vi "Controller Acquisition and Actuation Loop.vi"(4 "Iteration duration":u64, 5 "Missed iteration count":u32, 6 "Timestamp":u64, 7 "Sync Objects":T3, 8 "error in (no error)":errorcluster, 9 "PS Variables":T1, 10 "BPM Variables":T2, 11 "FOFB Configuration":T6={"FOFB Parameters"={"Network"={"FOFB Controller IP"="", "LNLS Control Network IP"="", "LNLS Control Network Power Supplies TCP Port"=0, "LNLS Control Network FOFB Configuration TCP Port"=0, "LNLS Control Network BPMs TCP Port"=0, "Data Server TCP Port"=0, "Monitoring Data TCP Port"=0, "Configuration GUI TCP Port"=0, "Storage Data TCP Port"=0, "Fast Command TCP Port"=0, "TCP Listening Timeout"=0, "Request Setpoints Rate"=0}, "Fast Acquisition"={"Acquisition Period"=0, "Data Buffer Size"=0, "Monitoring Period"=0}, "Response Matrix Measurement"={"Step Amplitude"=0.0, "Time Between Steps"=0, "Step Duration"=0, "Number of Averages"=0}, "Correction Algorithm"={"Correction Period"=0, "Reference Orbit Path"=path "", "Response Matrix Path"=path "", "Correction Matrix Path"=path "", "PID Horizontal Gain"=0.0, "PID Vertical Gain"=0.0, "PID Horizontal Integral Time"=0.0, "PID Vertical Integral Time"=0.0, "PID Horizontal Derivative Time"=0.0, "PID Vertical Derivative Time"=0.0, "Beam Current FOFB Threshold"=0.0, "Decouple H-V"=FALSE, "Use Additional BPM LPF"=FALSE, "BPM LPF Cutoff"=0.0}, "Acquisition Network"=[], "Actuation Network"=[]}, "Number of Acquisition Chassis"=0, "Number of Actuation Chassis"=0, "Number of BPM Readings"=0, "BPM Reading Names"=[], "Selected BPM Readings"=[0, 1, 2, 3, 4, 5, 6, 7, 8, 9, 10, 11, 12, 13, 14, 15, 16, 17, 18, 19, 20, 21, 22, 23, 24, 25, 26, 27, 28, 29, 30, 31, 32, 33, 34, 35, 36, 37, 38, 39, 40, 41, 42, 43, 44, 45, 46, 47, 48, 49], "Number of Correctors"=0, "Corrector Names"=[], "Selected Correctors"=[0, 1, 2, 3, 4, 5, 6, 7, 8, 9, 10, 11, 12, 13, 14, 15, 16, 17, 18, 19, 20, 21, 22, 23, 24, 25, 26, 27, 28, 29, 30, 31, 32, 33, 34, 35, 36, 37, 38, 39, 40, 41, 42, 43, 44, 45, 46, 47, 48, 49], "Reference Orbit"=[], "Response Matrix"=[], "Correction Matrix"=[], "Acquisition Chassis Names"=[], "Actuation Chassis Names"=[], "Acquisition Variables"=[], "Actuation Variables"=[], "PS Matrix Mapping"=[], "Inverse PS Matrix Mapping"=[], "BPM Matrix Mapping"=[], "Inverse BPM Matrix Mapping"=[], "Response Matrix Beam Energy (MeV)"=0.0, "PID Parameters"=[], "BPM Planes"=[], "Corrector Planes"=[], "RMM Step Factor"=[]}) -> (0 "error out":errorcluster)   [LabVIEW 2011, in "Controller VIs.lvlib"]
doc: "Continuously performs acquisition of all input variables (BPM readings, Power Supply readings, etc.) and forwards data to the <b>Decimated Acquisition Loop</b>. Depending on the <b>Actuation State</b> (global variable), performs actuations coming from one of the following sources (global variables):\n\n<b>Actuation State</b> = Only Reading\n (no actuation)\n\n<b>Actuation State</b> = Manual\n PS_Manual_Setpoints\n\n<b>Actuation State</b> = FOFB, Initializing FOFB, Stopping FOFB\n PS_FOFB_Setpoints\n\n<b>Actuation State</b> = Response Matrix Measurement\n PS_RMM_Setpoints"
uses:
  Controller VIs.lvlib
  Types Definitions/Type FOFB Configuration.ctl
  Types Definitions/Type FOFB Parameters.ctl
  Types Definitions/Type Network Configuration.ctl
  Types Definitions/Type FA Configuration.ctl
  Types Definitions/Type Response Matrix Measurement Configuration.ctl
  Types Definitions/Type Correction Algorithm Configuration.ctl
  Types Definitions/Type Acquisition Network Configuration.ctl
  Types Definitions/Type Actuation Network Configuration.ctl
  Types Definitions/Type PID Parameters.ctl
  Types Definitions/Type Synchronization Objects.ctl
  Types Definitions/Type Blocking Synchronization Objects.ctl
  Types Definitions/Type Monitoring Data.ctl
  Types Definitions/Type Operation Mode State.ctl
  Types Definitions/Type Diagnostics Data.ctl
  Types Definitions/Type CPU Loads Array.ctl
  Types Definitions/Type CPU Loads.ctl
  Types Definitions/Type Non-blocking Synchronization Objects.ctl
  Types Definitions/Type FOFB Variables.ctl
  Types Definitions/Type Actuation State.ctl
  Types Definitions/Type BPM Variables.ctl
  Types Definitions/Type PS Variables.ctl
  Controller Write FXP20.5.vi
  Controller Global Variables/Controller Actuation State.vi
  Type Definitions.lvlib
  Controller Global Variables.lvlib
panel:
  in  "Numeric":i32=3125
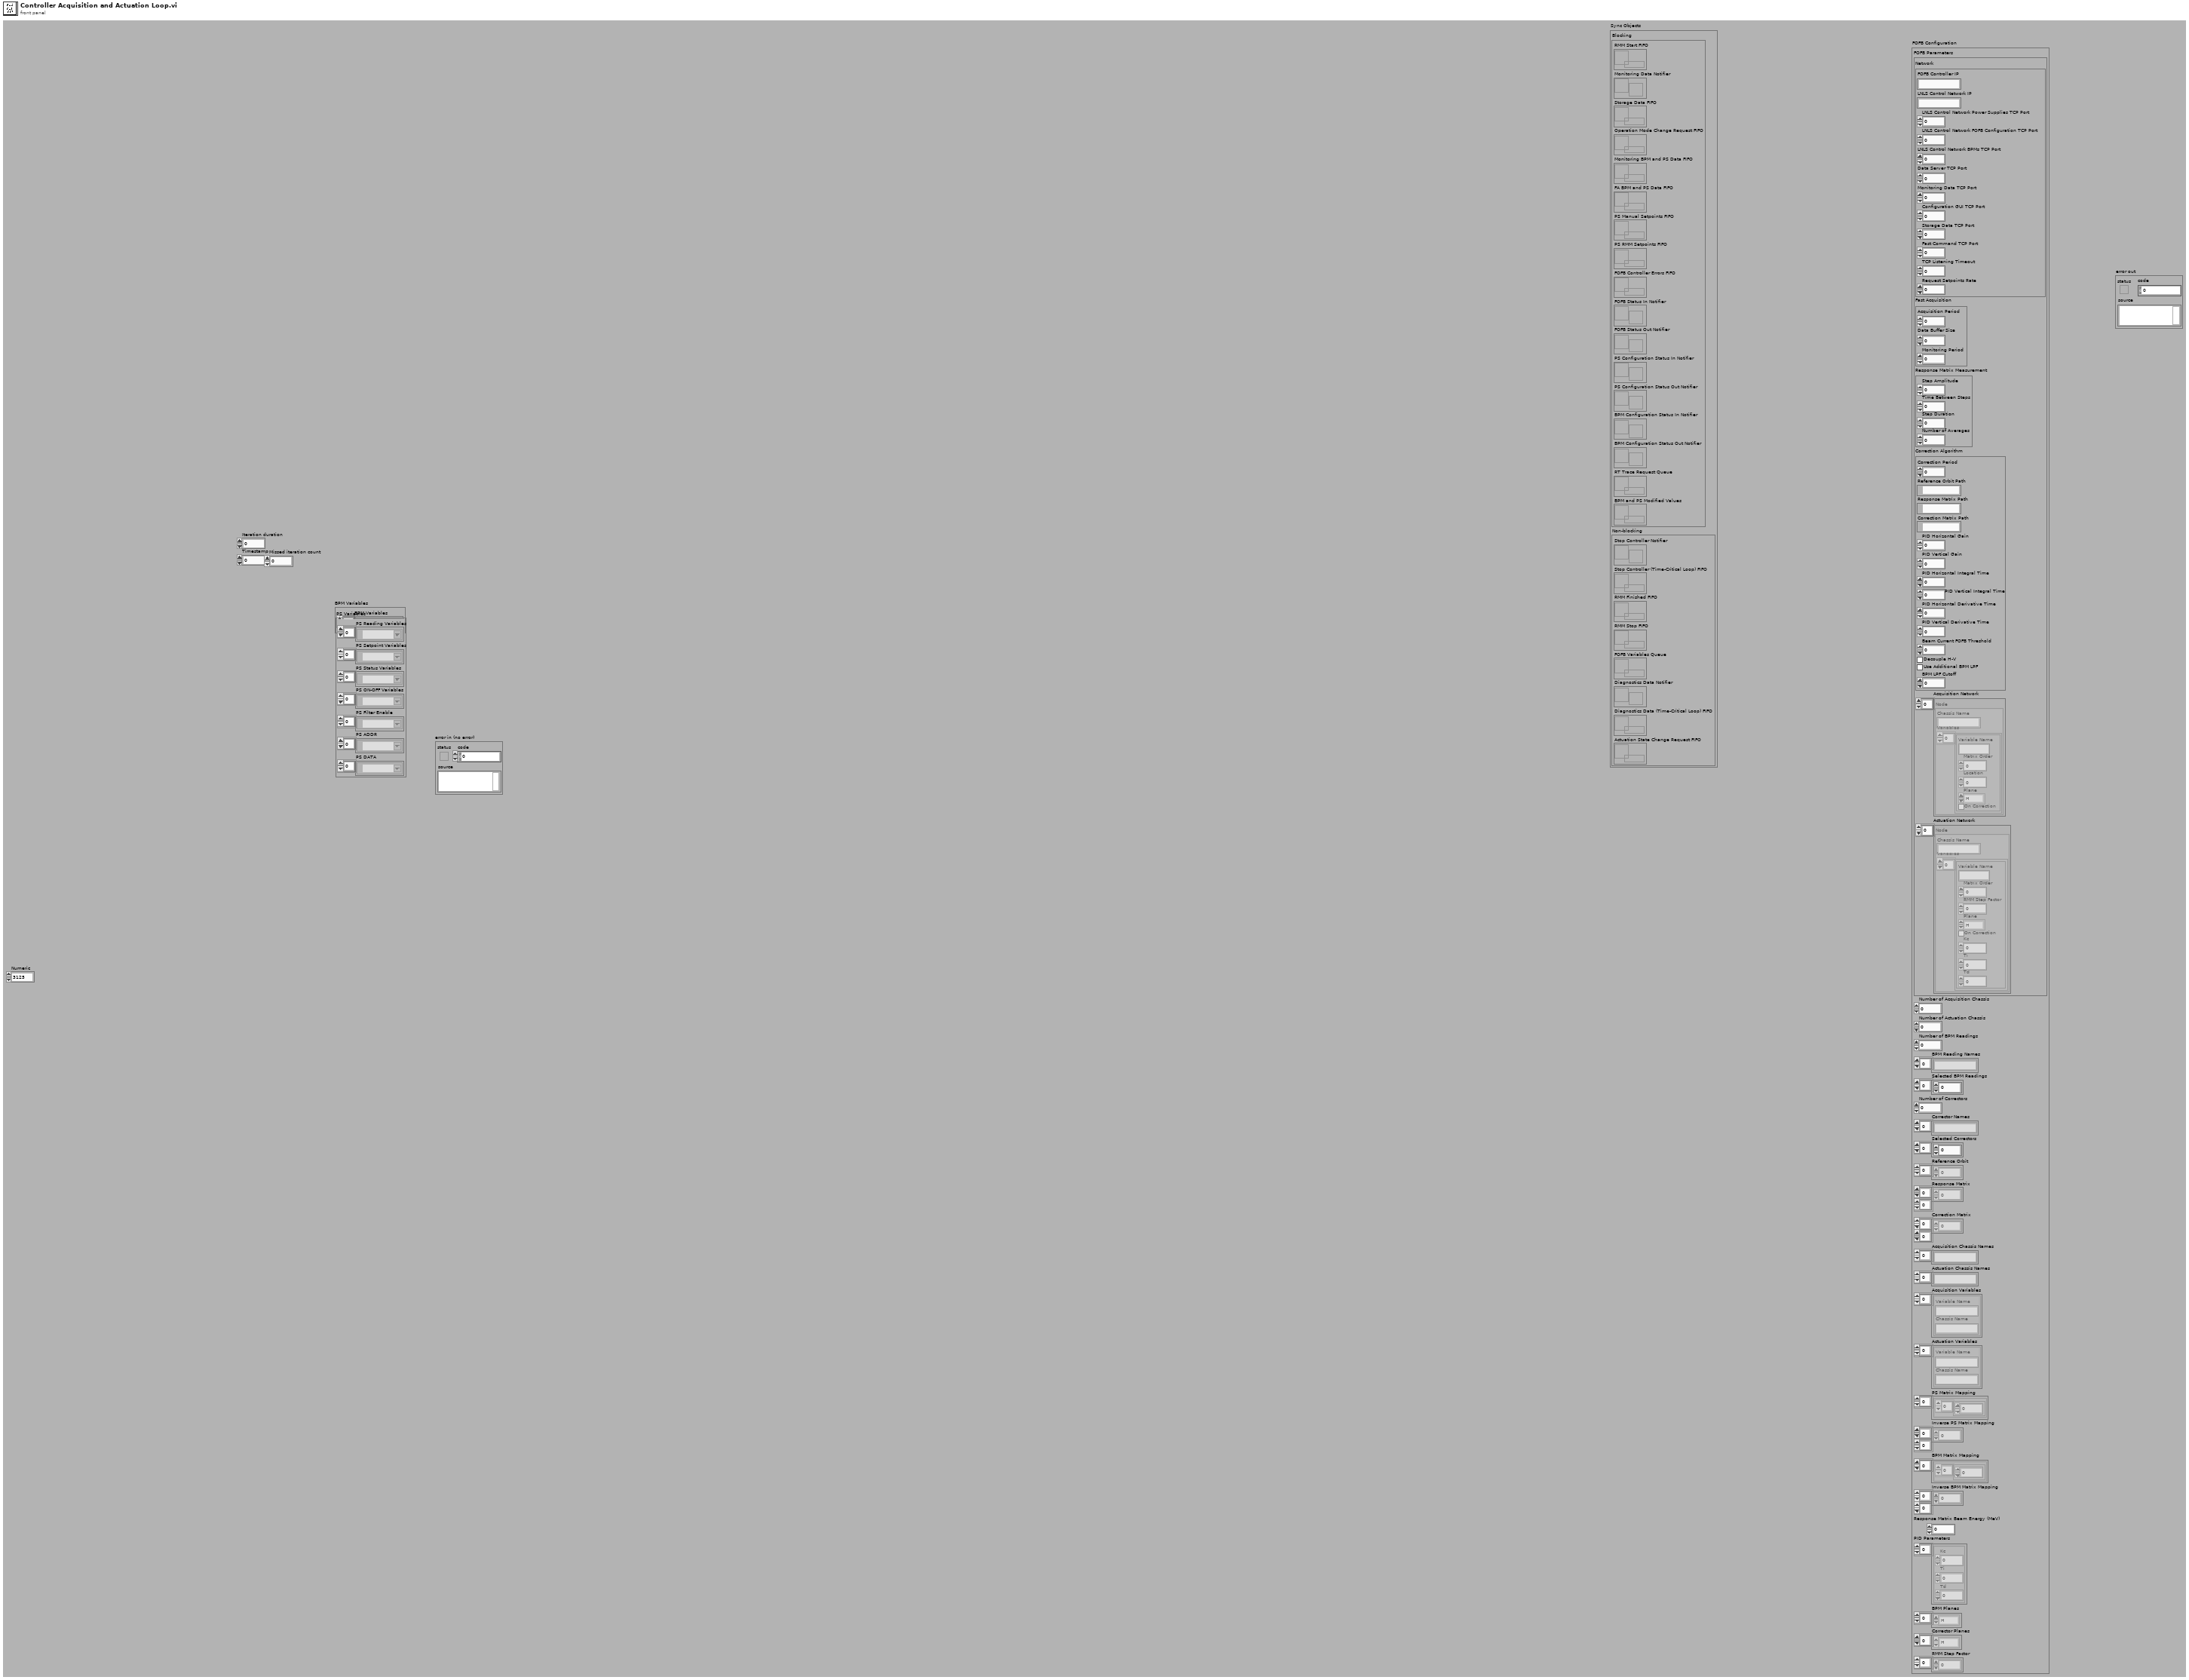
[diagram p1: front panel]
types:
  T1 = typedef "Type Definitions.lvlib/Type PS Variables.ctl" = cluster{"PS Reading Variables":refnum<k21>[], "PS Setpoint Variables":refnum<k21>[], "PS Status Variables":refnum<k21>[], "PS ON-OFF Variables":refnum<k21>[], "PS Filter Enable":refnum<k21>[], "PS ADDR":refnum<k21>[], "PS DATA":refnum<k21>[]}
  T2 = typedef "Type Definitions.lvlib/Type BPM Variables.ctl" = cluster{"BPM Variables":refnum<k21>[]}
  T3 = typedef "Type Definitions.lvlib/Type Synchronization Objects.ctl" = cluster{"Blocking":T4, "Non-blocking":T5}
  T4 = typedef "Type Definitions.lvlib/Type Blocking Synchronization Objects.ctl" = cluster{"RMM Start FIFO":refnum<k33>, "Monitoring Data Notifier":refnum<notifier>, "Storage Data FIFO":refnum<queue>, "Operation Mode Change Request FIFO":refnum<k33>, "Monitoring BPM and PS Data FIFO":refnum<k33>, "FA BPM and PS Data FIFO":refnum<k33>, "PS Manual Setpoints FIFO":refnum<k33>, "PS RMM Setpoints FIFO":refnum<k33>, "FOFB Controller Errors FIFO ":refnum<k33>, "FOFB Status In Notifier":refnum<notifier>, "FOFB Status Out Notifier":refnum<notifier>, "PS Configuration Status In Notifier":refnum<notifier>, "PS Configuration Status Out Notifier":refnum<notifier>, "BPM Configuration Status In Notifier":refnum<notifier>, "BPM Configuration Status Out Notifier":refnum<notifier>, "RT Trace Request Queue":refnum<queue>, "BPM and PS Modified Values":refnum<k33>}
  T5 = typedef "Type Definitions.lvlib/Type Non-blocking Synchronization Objects.ctl" = cluster{"Stop Controller Notifier":refnum<notifier>, "Stop Controller (Time-Critical Loop) FIFO":refnum<k33>, "RMM Finished FIFO":refnum<k33>, "RMM Stop FIFO":refnum<k33>, "FOFB Variables Queue":refnum<queue>, "Diagnostics Data Notifier":refnum<notifier>, "Diagnostics Data (Time-Critical Loop) FIFO":refnum<k33>, "Actuation State Change Request FIFO":refnum<k33>}
  T6 = typedef "Type Definitions.lvlib/Type FOFB Configuration.ctl" = cluster{"FOFB Parameters":T7, "Number of Acquisition Chassis":i32, "Number of Actuation Chassis":i32, "Number of BPM Readings":i32, "BPM Reading Names":string[], "Selected BPM Readings":u32[], "Number of Correctors":i32, "Corrector Names":string[], "Selected Correctors":u32[], "Reference Orbit":dbl[], "Response Matrix":dbl[][], "Correction Matrix":dbl[][], "Acquisition Chassis Names":string[], "Actuation Chassis Names":string[], "Acquisition Variables":cluster{"Variable Name":string, "Chassis Name":string}[], "Actuation Variables":cluster{"Variable Name":string, "Chassis Name":string}[], "PS Matrix Mapping":cluster{u32[]}[], "Inverse PS Matrix Mapping":u32[][], "BPM Matrix Mapping":cluster{u32[]}[], "Inverse BPM Matrix Mapping":u32[][], "Response Matrix Beam Energy (MeV)":dbl, "PID Parameters":T14[], "BPM Planes":enum8{"H", "V"}[], "Corrector Planes":enum8{"H", "V"}[], "RMM Step Factor":dbl[]}
  T7 = typedef "Type Definitions.lvlib/Type FOFB Parameters.ctl" = cluster{"Network":T8, "Fast Acquisition":T9, "Response Matrix Measurement":T10, "Correction Algorithm":T11, "Acquisition Network":T12, "Actuation Network":T13}
  T8 = typedef "Type Definitions.lvlib/Type Network Configuration.ctl" = cluster{"FOFB Controller IP":string, "LNLS Control Network IP":string, "LNLS Control Network Power Supplies TCP Port":u16, "LNLS Control Network FOFB Configuration TCP Port":u16, "LNLS Control Network BPMs TCP Port":u16, "Data Server TCP Port":u16, "Monitoring Data TCP Port":u16, "Configuration GUI TCP Port":u16, "Storage Data TCP Port":u16, "Fast Command TCP Port":u16, "TCP Listening Timeout":i32, "Request Setpoints Rate":u16}
  T9 = typedef "Type Definitions.lvlib/Type FA Configuration.ctl" = cluster{"Acquisition Period":u32, "Data Buffer Size":u32, "Monitoring Period":u32}
  T10 = typedef "Type Definitions.lvlib/Type Response Matrix Measurement Configuration.ctl" = cluster{"Step Amplitude":dbl, "Time Between Steps":u32, "Step Duration":u32, "Number of Averages":u32}
  T11 = typedef "Type Definitions.lvlib/Type Correction Algorithm Configuration.ctl" = cluster{"Correction Period":u32, "Reference Orbit Path":path, "Response Matrix Path":path, "Correction Matrix Path":path, "PID Horizontal Gain":dbl, "PID Vertical Gain":dbl, "PID Horizontal Integral Time":dbl, "PID Vertical Integral Time":dbl, "PID Horizontal Derivative Time":dbl, "PID Vertical Derivative Time":dbl, "Beam Current FOFB Threshold":dbl, "Decouple H-V":bool, "Use Additional BPM LPF":bool, "BPM LPF Cutoff":dbl}
  T12 = typedef "Type Definitions.lvlib/Type Acquisition Network Configuration.ctl" = cluster{"Chassis Name":string, "Variables":cluster{"Variable Name":string, "Matrix Order":u32, "Location":dbl, "Plane":enum8{"H", "V"}, "On Correction":bool}[]}[]
  T13 = typedef "Type Definitions.lvlib/Type Actuation Network Configuration.ctl" = cluster{"Chassis Name":string, "Variables":cluster{"Variable Name":string, "Matrix Order":u32, "RMM Step Factor":dbl, "Plane":enum8{"H", "V"}, "On Correction":bool, "Kc":dbl, "Ti":dbl, "Td":dbl}[]}[]
  T14 = typedef "Type Definitions.lvlib/Type PID Parameters.ctl" = cluster{"Kc":fxp<+/-,16,8>, "Ti":fxp<+/-,16,8>, "Td":fxp<+/-,16,8>}
  T15 = typedef "Type Definitions.lvlib/Type Actuation State.ctl" = enum8{"Only reading", "Manual", "FOFB Initialization", "FOFB", "FOFB Stopping", "RMM Initialization", "RMM", "RMM Stopping"}
  T16 = typedef "Type Definitions.lvlib/Type FOFB Variables.ctl" = cluster{"Correction Period":u32, "Reference Orbit":dbl[], "Response Matrix":dbl[][], "Correction Matrix":dbl[][], "Decouple H-V":bool, "PID Horizontal Gain":dbl, "PID Vertical Gain":dbl, "PID Horizontal Integral Time":dbl, "PID Vertical Integral Time":dbl, "PID Horizontal Derivative Time":dbl, "PID Vertical Derivative Time":dbl, "Selected BPM Readings":u32[], "Selected Correctors":u32[], "BPM Planes":enum8{"H", "V"}[], "Corrector Planes":enum8{"H", "V"}[], "Beam Current FOFB Threshold":dbl, "Response Matrix Beam Energy (MeV)":dbl, "Fast Command Enabled":bool}
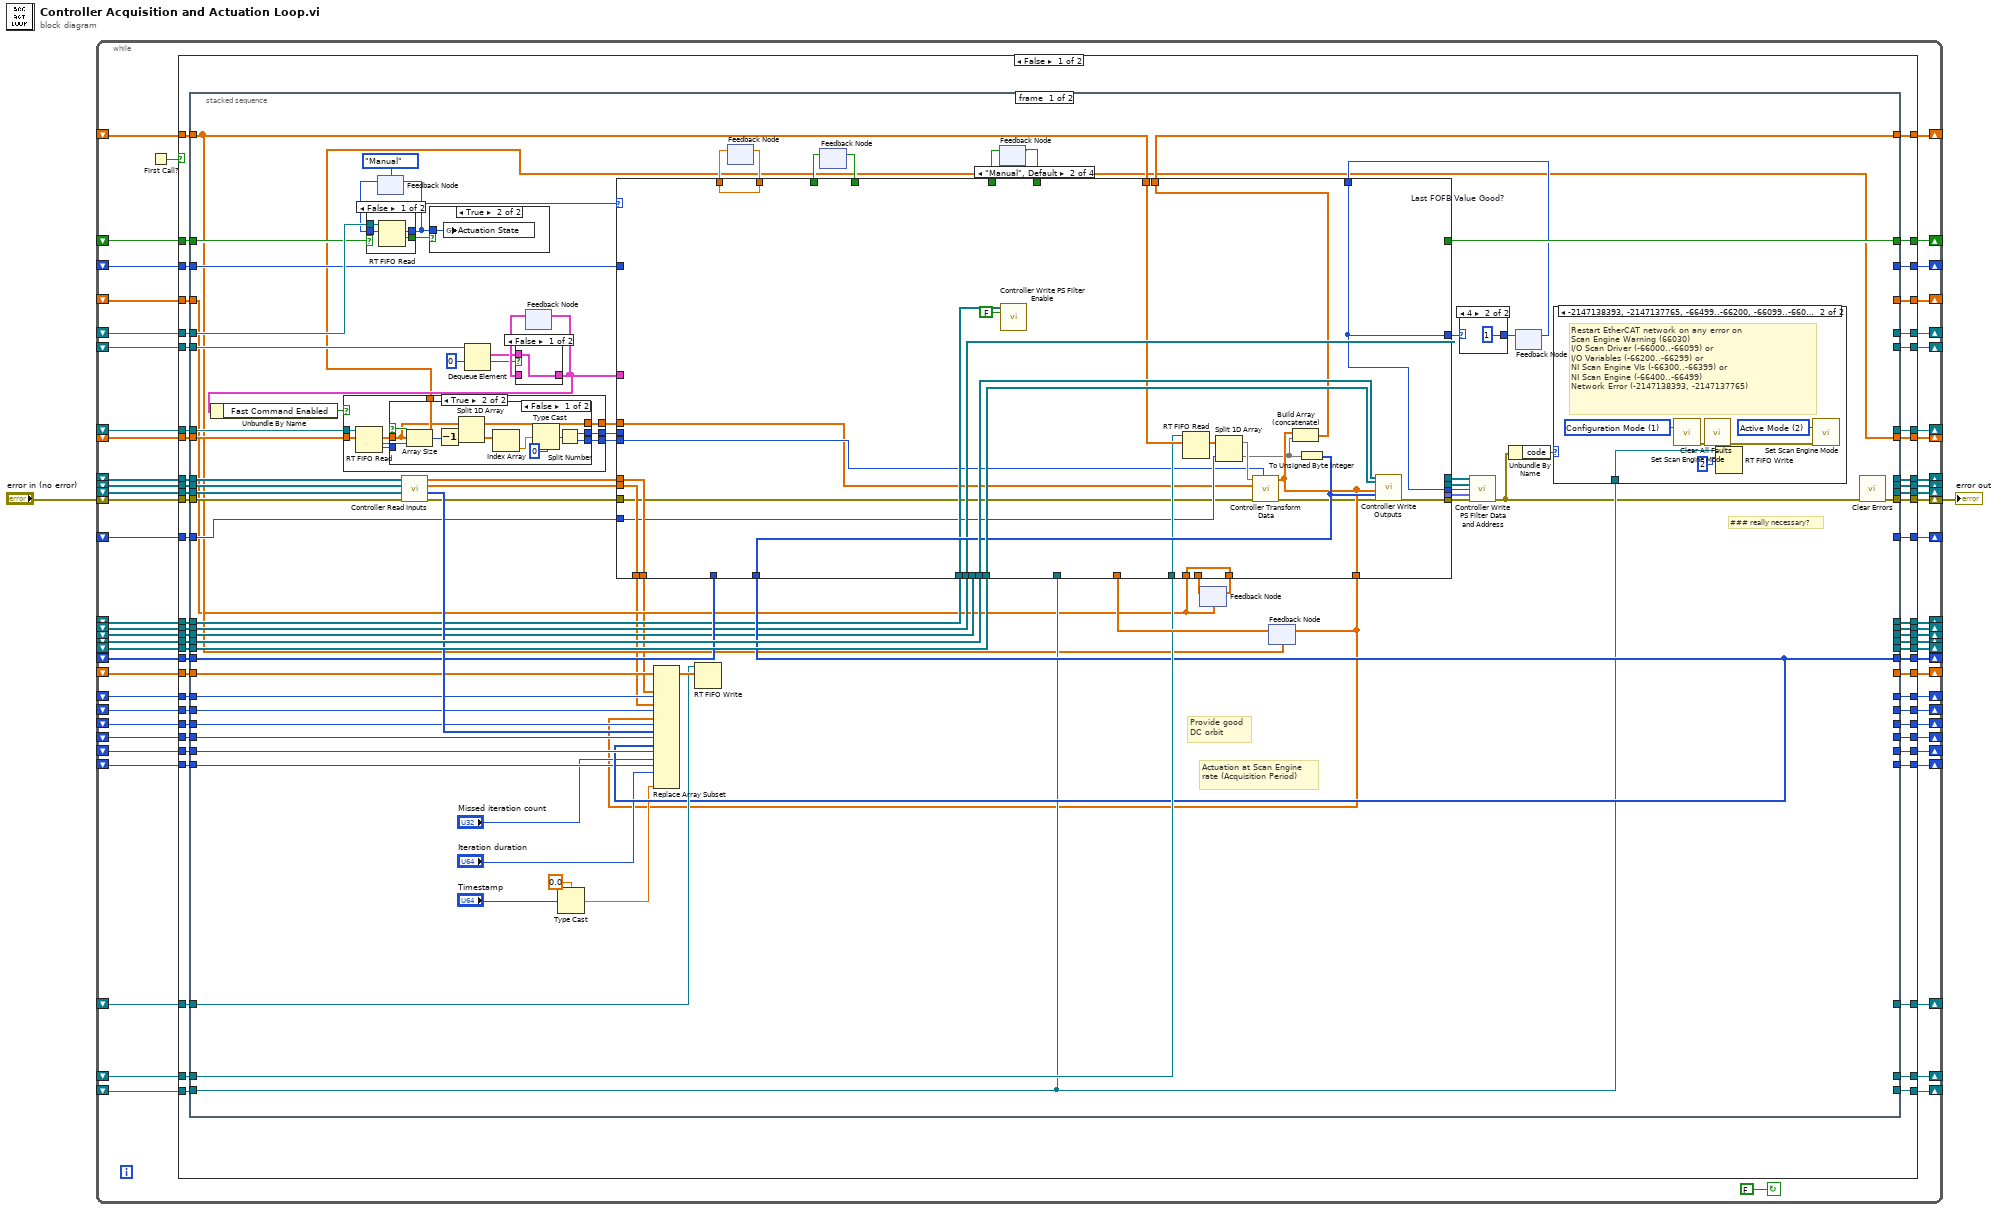
[diagram p0: block diagram]
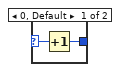
[diagram p3: hidden frame]
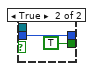
[diagram p4: hidden frame]
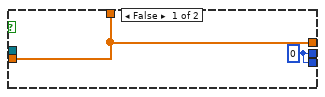
[diagram p5: hidden frame]
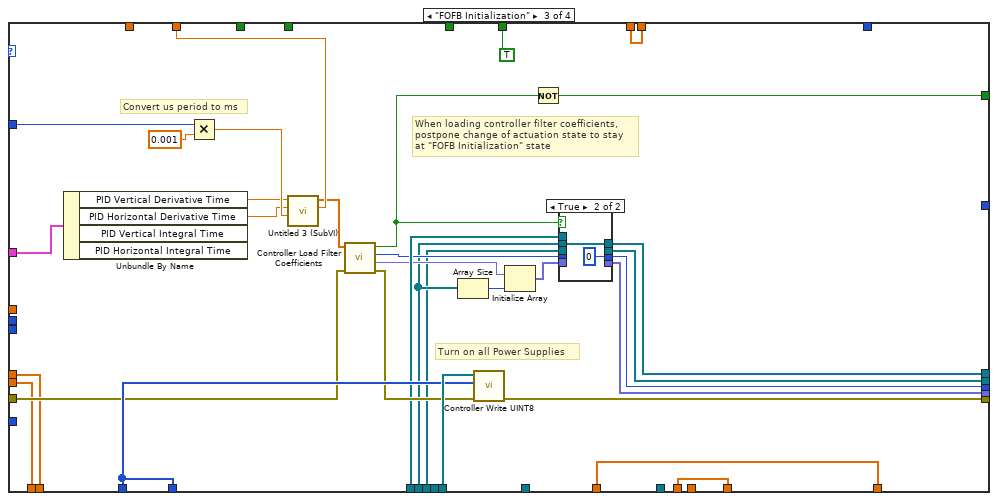
[diagram p10: hidden frame]
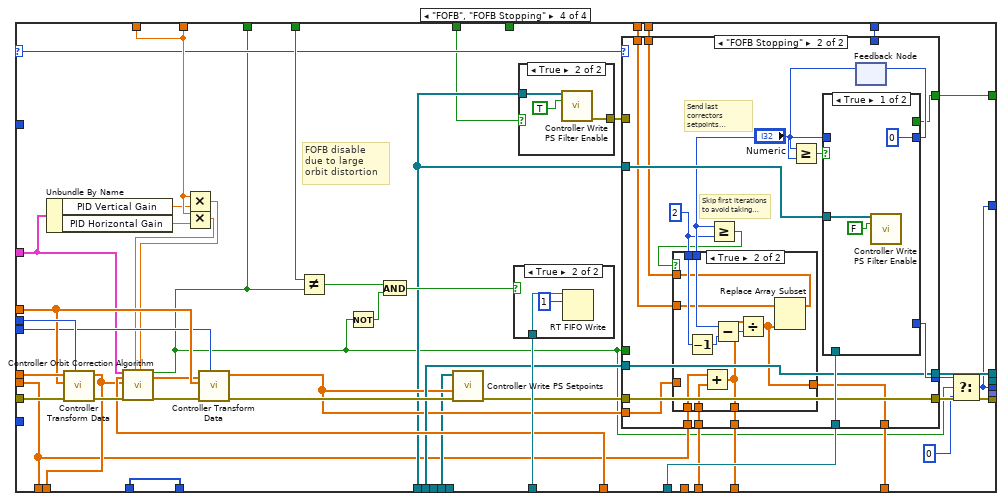
[diagram p12: hidden frame]
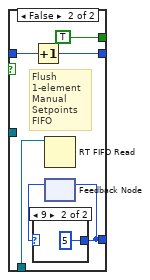
[diagram p15: hidden frame]
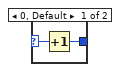
[diagram p16: hidden frame]
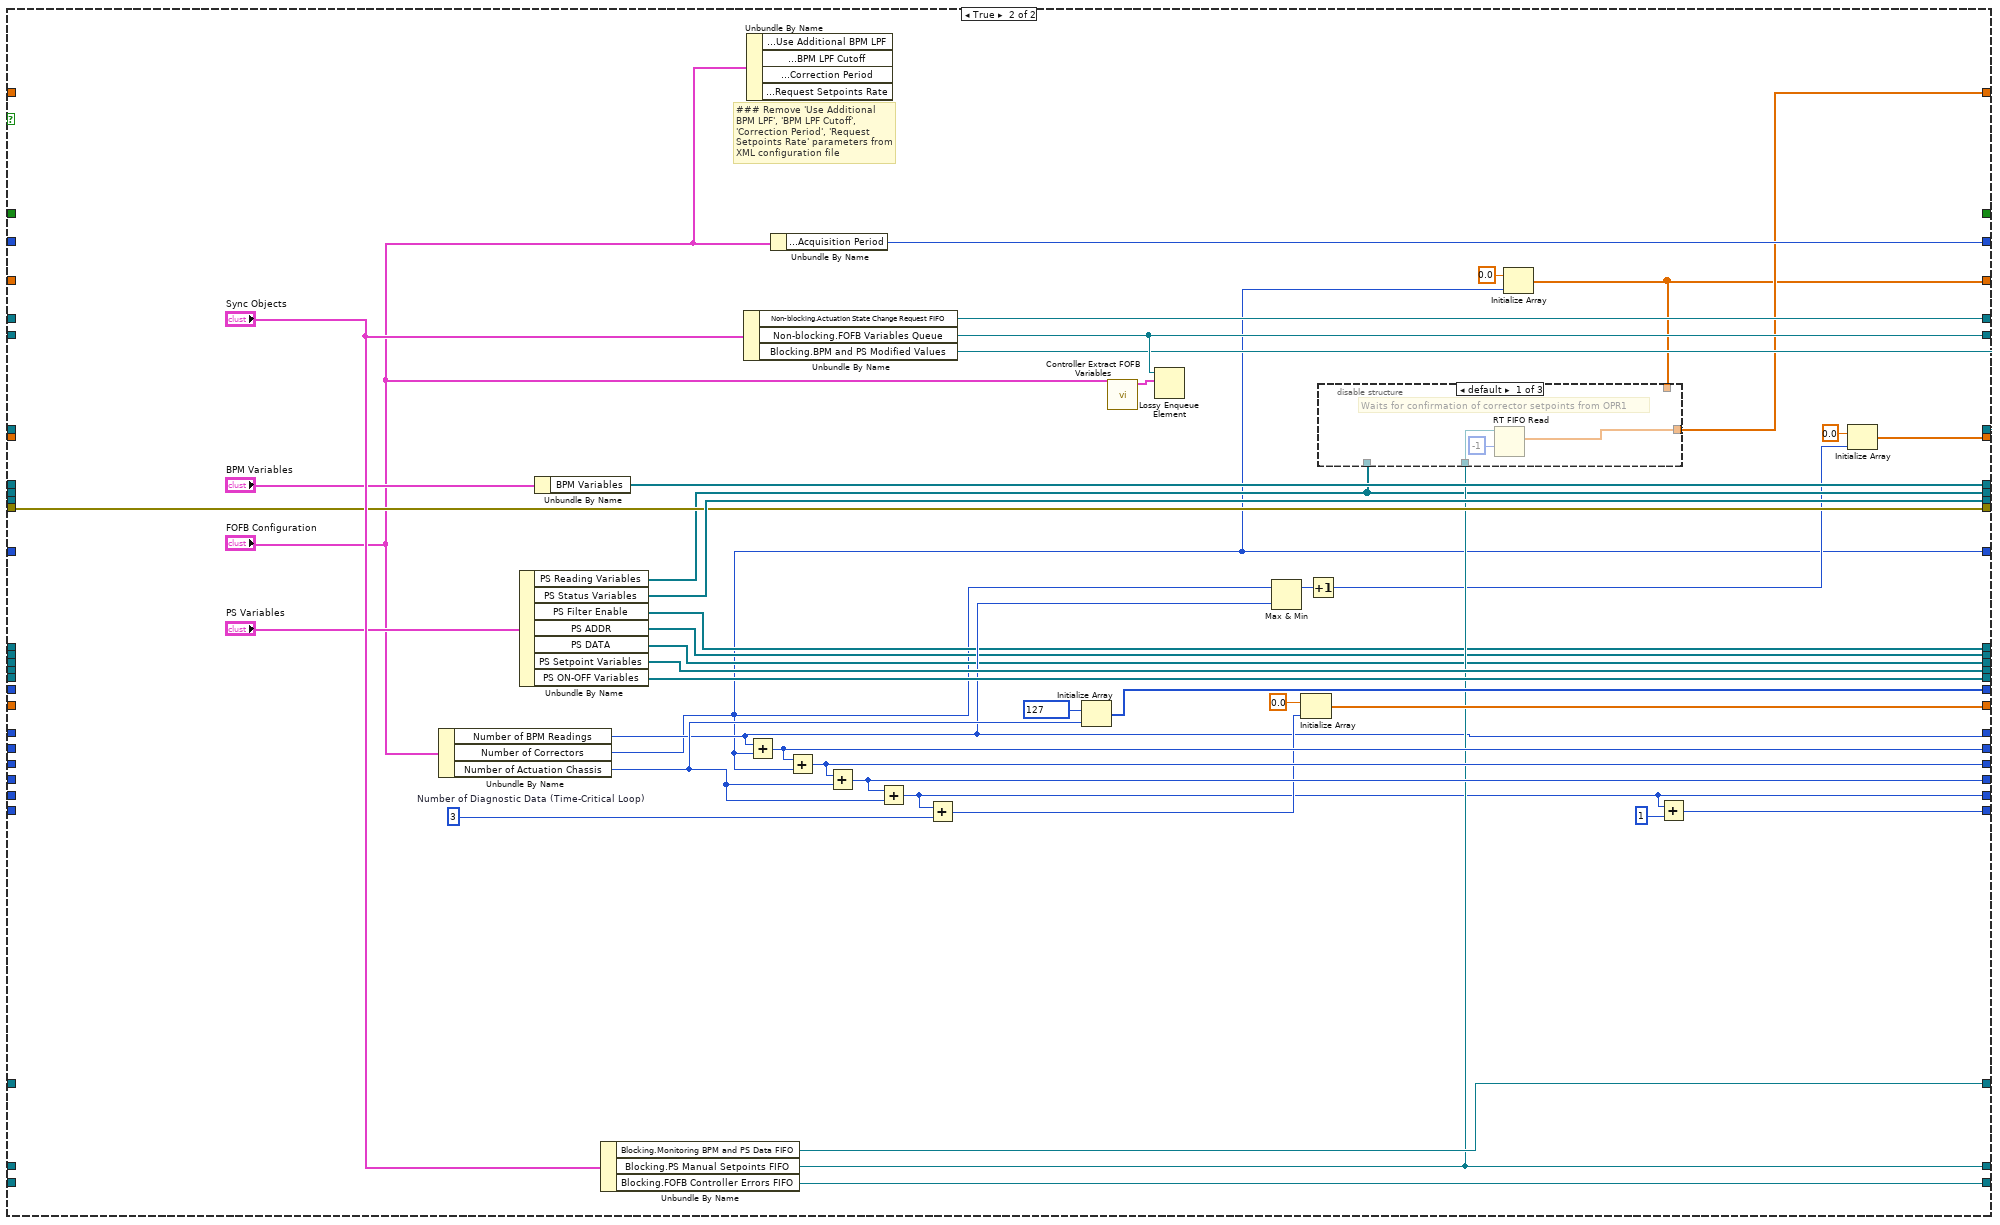
[diagram p20: hidden frame]
diagram:
  n1 = while {
    shift-right: [w49] -> w2
    shift-left: "error in (no error)" -> [w17]
    shift-right: [w45] -> _
    shift-left: _ -> [w57]
    shift-right: [w44] -> _
    shift-left: _ -> [w62]
    shift-right: [w43] -> _
    shift-left: _ -> [w61]
    shift-right: [w42] -> _
    shift-left: _ -> [w59]
    shift-right: [w41] -> _
    shift-left: _ -> [w48]
    shift-right: [w40] -> _
    shift-left: _ -> [w58]
    shift-right: [w39] -> _
    shift-left: _ -> [w56]
    shift-right: [w38] -> _
    shift-left: _ -> [w60]
    shift-right: [w37] -> _
    shift-left: _ -> [w53]
    shift-right: [w36] -> _
    shift-left: _ -> [w55]
    shift-right: [w35] -> _
    shift-left: _ -> [w52]
    shift-right: [w34] -> _
    shift-left: _ -> [w54]
    shift-right: [w33] -> _
    shift-left: _ -> [w51]
    shift-right: [w32] -> _
    shift-left: _ -> [w50]
    shift-right: [w31] -> _
    shift-left: _ -> [w28]
    shift-right: [w30] -> _
    shift-left: _ -> [w27]
    shift-right: [w29] -> _
    shift-left: _ -> [w26]
    shift-right: [w24] -> _
    shift-left: _ -> [w25]
    shift-right: [w22] -> _
    shift-left: _ -> [w23]
    shift-right: [w21] -> _
    shift-left: _ -> [w20]
    shift-right: [w19] -> _
    shift-left: _ -> [w18]
    shift-right: [w14] -> _
    shift-left: _ -> [w15]
    shift-right: [w13] -> _
    shift-left: _ -> [w16]
    shift-right: [w11] -> _
    shift-left: _ -> [w12]
    shift-right: [w9] -> _
    shift-left: _ -> [w10]
    shift-right: [w7] -> _
    shift-left: _ -> [w6]
    shift-right: [w8] -> _
    shift-left: _ -> [w5]
    shift-right: [w4] -> _
    shift-left: _ -> [w3]
    stop <- FALSE continue-if-true
    n2 = First Call?() -> (First Call?: T/F=w46:bool)
    n3 = case shown="False" w46 {
      tunnel: w62 -> [w120 _]
      tunnel: w61 -> [w119 _]
      tunnel: w60 -> [w118 _]
      tunnel: w59 -> [w117 _]
      tunnel: w58 -> [w116 _]
      tunnel: w57 -> [w115 _]
      tunnel: w56 -> [w114 _]
      tunnel: w55 -> [w113 _]
      tunnel: w54 -> [w112 _]
      tunnel: w53 -> [w111 _]
      tunnel: w52 -> [w110 _]
      tunnel: w51 -> [w109 _]
      tunnel: w50 -> [w108 _]
      tunnel: [w107 w458] -> w49
      tunnel: w17 -> [w106 w458]
      tunnel: w48 -> [w105 _]
      tunnel: [w103 w476] -> w45
      tunnel: [w102 w475] -> w44
      tunnel: [w101 w454] -> w43
      tunnel: [w100 w474] -> w42
      tunnel: [w99 w435] -> w41
      tunnel: [w98 w473] -> w40
      tunnel: [w97 w440] -> w39
      tunnel: [w96 w472] -> w38
      tunnel: [w95 w471] -> w37
      tunnel: [w94 w444] -> w36
      tunnel: [w93 w470] -> w35
      tunnel: [w92 w469] -> w34
      tunnel: [w91 w468] -> w33
      tunnel: [w90 w450] -> w32
      tunnel: [w83 w461] -> w31
      tunnel: [w82 w455] -> w30
      tunnel: [w81 w460] -> w29
      tunnel: w28 -> [w85 _]
      tunnel: w27 -> [w84 _]
      tunnel: w26 -> [w104 _]
      tunnel: w25 -> [w89 _]
      tunnel: [w88 w459] -> w24
      tunnel: w23 -> [w87 _]
      tunnel: [w86 w437] -> w22
      tunnel: w20 -> [w80 _]
      tunnel: [w79 w456] -> w21
      tunnel: [w77 w452] -> w19
      tunnel: w18 -> [w78 _]
      tunnel: w16 -> [w76 _]
      tunnel: w15 -> [w75 _]
      tunnel: [w74 w448] -> w14
      tunnel: [w73 w443] -> w13
      tunnel: w12 -> [w72 _]
      tunnel: [w71 _] -> w11
      tunnel: w10 -> [w70 _]
      tunnel: [w69 w441] -> w9
      tunnel: [w66 w439] -> w8
      tunnel: [w65 w438] -> w7
      tunnel: w6 -> [w68 _]
      tunnel: w5 -> [w67 _]
      tunnel: [w63 w434] -> w4
      tunnel: w3 -> [w64 _]
      frame False {
        n4 = stacked-sequence {
          tunnel: w120 -> [w199 w432]
          tunnel: w119 -> [w198 w431]
          tunnel: w118 -> [w197 w426]
          tunnel: w117 -> [w196 w430]
          tunnel: w116 -> [w194 w428]
          tunnel: w115 -> [w193 w433]
          tunnel: w114 -> [w147 w427]
          tunnel: w113 -> [w191 w424]
          tunnel: w112 -> [w190 w422]
          tunnel: w111 -> [w189 w425]
          tunnel: w110 -> [w186 w423]
          tunnel: w109 -> [w185 w421]
          tunnel: w108 -> [w184 w420]
          tunnel: [w170 _] -> w107
          tunnel: w106 -> [w182 _]
          tunnel: w105 -> [w171 w429]
          tunnel: w85 -> [w181 w419]
          tunnel: w104 -> [w174 w417]
          tunnel: w84 -> [w180 w418]
          tunnel: [_ w433] -> w103
          tunnel: [_ w432] -> w102
          tunnel: [_ w431] -> w101
          tunnel: [_ w430] -> w100
          tunnel: [_ w429] -> w99
          tunnel: [_ w428] -> w98
          tunnel: [_ w427] -> w97
          tunnel: [_ w426] -> w96
          tunnel: [_ w425] -> w95
          tunnel: [_ w424] -> w94
          tunnel: [_ w423] -> w93
          tunnel: [_ w422] -> w92
          tunnel: [_ w421] -> w91
          tunnel: [_ w420] -> w90
          tunnel: [_ w419] -> w83
          tunnel: [_ w418] -> w82
          tunnel: [_ w417] -> w81
          tunnel: w89 -> [w179 _]
          tunnel: [w178 _] -> w88
          tunnel: w87 -> [w133 _]
          tunnel: [w177 _] -> w86
          tunnel: w80 -> [w176 w416]
          tunnel: [_ w416] -> w79
          tunnel: w78 -> [w175 w415]
          tunnel: [_ w415] -> w77
          tunnel: w76 -> [w163 w414]
          tunnel: w75 -> [w158 _]
          tunnel: [w129 _] -> w74
          tunnel: [_ w414] -> w73
          tunnel: w72 -> [w154 _]
          tunnel: [w153 _] -> w71
          tunnel: w70 -> [w150 w413]
          tunnel: [_ w413] -> w69
          tunnel: w68 -> [w149 w411]
          tunnel: w67 -> [w148 w412]
          tunnel: [_ w412] -> w66
          tunnel: [_ w411] -> w65
          tunnel: w64 -> [w130 w410]
          tunnel: [_ w410] -> w63
          frame #0 {
            # "Actuation at Scan Engine rate (Acquisition Period)"
            # "Provide good\nDC orbit"
            # "### really necessary?"
            n5 = feedback #1(Type_Actuation_State."Manual" ("Actuation State")) -> (w137:T15)
            n6 = case shown="False" w154 {
              tunnel: w193 -> [w207 _]
              tunnel: w137 -> [w206 w209]
              tunnel: [w205 w209] -> w128
              tunnel: [w204 TRUE ("empty?")] -> w134
              frame False {
                n7 = RT FIFO Read(0:w207, 1:w206) -> (9:w205:T15, 10:w204:bool)  [unwired: 2 in, 3 out]
              }
              frame True {
              }
            }
            n8 = feedback-in #1(w128) -> ()
            n9 = call "Controller Read Inputs.vi"("error in (no error)"=w182, "PS Status Variables"=w196, "PS Reading Variables"=w198, "BPM Variables"=w199) -> ("error out"=w162:errorcluster, "PS Status (per PS Rack)"=w192:u8[], "PS Readings"=w125:dbl[], "BPM Readings"=w127:dbl[])  [unwired: 4 in]
            n10 = case shown="True" w134 {
              tunnel: w128 -> [_ w200]
              frame False {
              }
              frame True {
                n11 = global write "Controller Actuation State.vi" "Actuation State"(w200) -> ()
              }
            }
            n12 = Dequeue Element(queue=w175, timeout in ms (-1)=0) -> (element=w157:T16, timed out?=w164:bool)  [unwired: 1 in, 2 out]
            n13 = feedback #2() -> (w165:T16)  [unwired: 1 in]
            n14 = case shown="False" w164 {
              tunnel: [w230 w231] -> w155
              tunnel: w157 -> [w230 _]
              tunnel: w165 -> [_ w231]
              frame False {
              }
              frame True {
              }
            }
            n15 = Unbundle By Name(w155) -> ("Fast Command Enabled"=w156:bool)
            n16 = case shown="True" w156 {
              tunnel: w163 -> [_ w219]
              tunnel: [w211 w218] -> w161
              tunnel: [w210 w217] -> w160
              tunnel: [w210 w216] -> w159
              tunnel: w158 -> [w211 w215]
              tunnel: [w211 w214] -> w129
              frame False {
                w210 = u16 0
              }
              frame True {
                n17 = RT FIFO Read(0:w219, 1:w215) -> (7:w213:u32, 9:w214:sgl[], 10:w212:bool)  [unwired: 2 in, 2 out]
                n18 = case shown="False" w212 {
                  tunnel: [w228 _] -> w218
                  tunnel: [w224 _] -> w217
                  tunnel: [w223 _] -> w216
                  tunnel: w214 -> [w222 _]
                  tunnel: w213 -> [_ _]
                  frame False {
                    n19 = Array Size(array=w222) -> (size(s)=w229:i32)
                    n20 = Decrement(x=w229) -> (x-1=w227:i32)
                    n21 = Split 1D Array(array=w222, index=w227) -> (first subarray=w228:sgl[], second subarray=w221:sgl[])
                    n22 = Index Array(array=w221) -> (element=w220:sgl)  [unwired: 1 in]
                    n23 = Type Cast(type=u32 0, x=w220) -> (*(type *) &x=w225:u32)
                    n24 = Split Number(x=w225) -> (hi(x)=w224:u16, lo(x)=w223:u16)
                  }
                  frame True {
                  }
                }
              }
            }
            n25 = feedback-in #2(w155) -> ()
            n26 = Type Cast(type=0.0 ("double precision float"), x="Timestamp") -> (*(type *) &x=w173:dbl)
            n27 = feedback #3() -> (w151:dbl)  [unwired: 1 in]
            n28 = feedback #4 "Last FOFB Value Good?"() -> (w135:bool)  [unwired: 1 in]
            n29 = feedback #5() -> (w121:bool)  [unwired: 1 in]
            n30 = feedback #6(w130) -> (w131:dbl[])
            n31 = feedback #7(w133) -> (w195:dbl[])
            n32 = feedback #8() -> (w138:u8)  [unwired: 1 in]
            n33 = case shown="\"Manual\", Default" w128 {
              selector: w128 -> [_ _ _ w331]
              tunnel: [w246 w268 w302 w329] -> w146
              tunnel: w162 -> [w246 w249 w298 w354]
              tunnel: w127 -> [w240 w260 w274 w353]
              tunnel: w194 -> [_ w270 _ w323]
              tunnel: w197 -> [_ w269 w301 _]
              tunnel: w195 -> [w238 _ w272 w333]
              tunnel: w171 -> [_ w257 _ _]
              tunnel: w180 -> [_ w258 _ w321]
              tunnel: [w245 w267 w299 w352] -> w178
              tunnel: w179 -> [w245 _ w299 w352]
              tunnel: w155 -> [_ _ w285 w342]
              tunnel: [w244 w253 w300 w320] -> w177
              tunnel: w133 -> [w244 w262 w300 w319]
              tunnel: w174 -> [_ _ _ w337]
              tunnel: w161 -> [_ w252 _ w350]
              tunnel: w160 -> [_ _ _ w351]
              tunnel: w159 -> [_ w254 _ w349]
              tunnel: [_ _ w296 w324] -> w153
              tunnel: w125 -> [w239 w259 w273 w315]
              tunnel: [w243 w266 w284 w340] -> w152
              tunnel: w151 -> [w243 w266 _ w340]
              tunnel: w150 -> [_ _ w286 _]
              tunnel: w149 -> [_ w264 w294 w322]
              tunnel: w148 -> [w242 w263 w289 w328]
              tunnel: w147 -> [_ _ w288 _]
              tunnel: [_ _ w279 _] -> w144
              tunnel: [_ w247 w278 w311] -> w143
              tunnel: [_ _ w277 _] -> w142
              tunnel: [w242 w263 w276 w327] -> w141
              tunnel: w138 -> [_ w247 _ w336]
              tunnel: [_ w247 _ w311] -> w140
              tunnel: [_ _ _ w310] -> w136
              tunnel: w135 -> [_ _ _ w335]
              tunnel: [w241 w261 w275 w318] -> w132
              tunnel: w131 -> [_ _ _ w317]
              tunnel: w130 -> [w241 w261 w275 _]
              tunnel: [w240 w260 w274 w316] -> w126
              tunnel: [w239 w259 w273 w315] -> w124
              tunnel: [w238 w251 w272 w314] -> w123
              tunnel: [_ _ TRUE _] -> w122
              tunnel: w121 -> [_ _ _ w313]
              frame "Only reading" {
              }
              frame "Manual", Default {
                n34 = call "Controller Write PS Filter Enable.vi"("PS Filter Enable"=w264, "Filter Enable"=FALSE) -> ()  [unwired: 13 in, 1 out]
                n35 = RT FIFO Read(0:w258, 1:w262) -> (9:w255:dbl[])  [unwired: 2 in, 4 out]
                n36 = Split 1D Array(array=w255, index=w257) -> (first subarray=w256:dbl[], second subarray=w250:dbl[])
                n37 = call "Controller Transform Data.vi"("Mode (Transparent)"=w254, "error in (no error)"=w249, "New Data"=w252, "Data"=w256) -> ("error out"=w248:errorcluster, "Transformed Data"=w251:dbl[])  [unwired: 6 in]
                n38 = Build Array (concatenate)(w251, w250) -> (w253:dbl[])
                n39 = To Unsigned Byte Integer(number=w250) -> (unsigned 8bit integer=w267:u8[])
                n40 = call "Controller Write Outputs.vi"("PS Setpoint Variables"=w270, "PS ON-OFF Variables"=w269, "PS Setpoints"=w251, "PS ON-OFF (per PS Rack)"=w267, "error in (no error)"=w248) -> ("error out"=w268:errorcluster)  [unwired: 14 in]
              }
              frame "FOFB Initialization" {
                # "Convert us period to ms"
                # "When loading controller filter coefficients,\npostpone change of actuation state to stay\nat \"FOFB Initialization\" state"
                # "Turn on all Power Supplies"
                n41 = Unbundle By Name(w285) -> ("PID Vertical Derivative Time"=w281:dbl, "PID Horizontal Derivative Time"=w280:dbl)  [unwired: 2 out]
                n42 = Multiply(x=w286, y=0.001) -> (x*y=w282:dbl)
                n43 = call "Untitled 3 (SubVI).vi"("Period"=w282, "Derivative Time"=w280, "Integral Time"=w281) -> ("Scaling Gain"=w284:dbl, "PS Filter Coefficients"=w283:dbl[])  [unwired: 7 in]
                n44 = call "Controller Load Filter Coefficients.vi"("error in (no error)"=w298, "Coefficients"=w283) -> ("error out"=w297:errorcluster, "Data"=w292:fxp<+/-,20,2>, "Address"=w293:u8, "All coefficients loaded?"=w295:bool)  [unwired: 6 in]
                n45 = Array Size(array=w289) -> (size(s)=w291:i32)
                n46 = call "Controller Write UINT8.vi"("error in (no error)"=w297, "Values"=w299, "Variables"=w301) -> ("error out"=w302:errorcluster)  [unwired: 8 in]
                n47 = Initialize Array(w292, w291) -> (w290:fxp<+/-,20,2>[])
                n48 = Not(x=w295) -> (.not. x?=w296:bool)
                n49 = case shown="True" w295 {
                  tunnel: w289 -> [w303 w308]
                  tunnel: w294 -> [_ _]
                  tunnel: w293 -> [w305 _]
                  tunnel: w290 -> [w306 _]
                  tunnel: w288 -> [w304 _]
                  tunnel: [w306 _] -> w279
                  tunnel: [w305 u8 0 ("Address")] -> w278
                  tunnel: [w304 _] -> w277
                  tunnel: [w303 w308] -> w276
                  frame False {
                  }
                  frame True {
                  }
                }
              }
              frame "FOFB", "FOFB Stopping" {
                # "FOFB disable\ndue to large\norbit distortion"
                n50 = Unbundle By Name(w342) -> ("PID Vertical Gain"=w332:dbl, "PID Horizontal Gain"=w341:dbl)
                n51 = call "Controller Transform Data.vi"("Mode (Transparent)"=w351, "error in (no error)"=w354, "New Data"=w350, "Data"=w353) -> ("error out"=w346:errorcluster, "Transformed Data"=w316:dbl[])  [unwired: 6 in]
                n52 = Multiply(x=w340, y=w332) -> (x*y=w339:dbl)
                n53 = Multiply(x=w340, y=w341) -> (x*y=w338:dbl)
                n54 = call "Controller Orbit Correction Algorithm.vi"("FOFB Variables"=w342, "Corrector Kick Vector in"=w333, "Beam Position Vector"=w316, "error in (no error)"=w346, "Horizontal Gain"=w338, "Vertical Gain"=w339) -> ("Good value?"=w310:bool, "Corrector Kick Vector out"=w343:dbl[], "error out"=w345:errorcluster)  [unwired: 11 in]
                n55 = call "Controller Transform Data.vi"("Mode (Transparent)"=w349, "error in (no error)"=w345, "New Data"=w350, "Data"=w343) -> ("error out"=w344:errorcluster, "Transformed Data"=w326:dbl[])  [unwired: 6 in]
                n56 = Not Equal?(x=w335, y=w310) -> (x != y?=w334:bool)
                n57 = Not(x=w310) -> (.not. x?=w347:bool)
                n58 = And(x=w334, y=w347) -> (x .and. y?=w348:bool)
                n59 = call "Controller Write PS Setpoints.vi"("PS Setpoint Variables"=w323, "PS Setpoints"=w326, "error in (no error)"=w344) -> ("error out"=w330:errorcluster)  [unwired: 7 in]
                n60 = case shown="True" w348 {
                  tunnel: w337 -> [_ w408]
                  frame False {
                  }
                  frame True {
                    n61 = RT FIFO Write(0:w408, 1:u16 1 ("element")) -> ()  [unwired: 3 in, 4 out]
                  }
                }
                n62 = case shown="True" w313 {
                  tunnel: w322 -> [_ w406]
                  tunnel: [_ w405] -> w325
                  frame False {
                  }
                  frame True {
                    n63 = call "Controller Write PS Filter Enable.vi"("PS Filter Enable"=w406, "Filter Enable"=TRUE) -> ("error out"=w405:errorcluster)  [unwired: 13 in]
                  }
                }
                n64 = case shown="\"FOFB Stopping\"" w331 {
                  tunnel: w336 -> [w355 _]
                  tunnel: [w355 w374] -> w312
                  tunnel: w310 -> [_ _]
                  tunnel: w330 -> [w360 w369]
                  tunnel: [w360 w369] -> w329
                  tunnel: w328 -> [w357 w370]
                  tunnel: [w357 w370] -> w327
                  tunnel: [w359 w364] -> w314
                  tunnel: w315 -> [_ w373]
                  tunnel: w326 -> [w359 w363]
                  tunnel: w325 -> [_ _]
                  tunnel: [_ w361] -> w324
                  tunnel: w322 -> [_ w378]
                  tunnel: w321 -> [_ w375]
                  tunnel: [w358 w365] -> w320
                  tunnel: w319 -> [w358 w366]
                  tunnel: [w356 w371] -> w318
                  tunnel: w317 -> [w356 w372]
                  frame "FOFB", Default {
                  }
                  frame "FOFB Stopping" {
                    w367 = 2 ("y")
                    # "Skip first iterations\nto avoid taking\nPS reading values\ninstead of PS\nsetpoint values"
                    # "Send last correctors setpoints \nto next operation mode"
                    n65 = feedback #9() -> (w368:i32)  [unwired: 1 in]
                    n66 = Greater Or Equal?(x=w368, y=w367) -> (x >= y?=w362:bool)
                    n67 = case shown="True" w362 {
                      tunnel: w373 -> [_ w392]
                      tunnel: w372 -> [w382 w391]
                      tunnel: [w382 w390] -> w371
                      tunnel: w368 -> [_ w388]
                      tunnel: w367 -> [_ w389]
                      tunnel: w366 -> [w381 w385]
                      tunnel: [w381 w384] -> w365
                      tunnel: [w380 w383] -> w364
                      tunnel: w363 -> [w380 _]
                      frame False {
                      }
                      frame True {
                        n68 = Decrement(x=w389) -> (x-1=w386:i32)
                        n69 = Add(x=w392, y=w391) -> (x+y=w390:dbl[])
                        n70 = Subtract(x=w388, y=w386) -> (x-y=w387:i32)
                        n71 = Divide(x=w390, y=w387) -> (x/y=w383:dbl[])
                        n72 = Replace Array Subset(array=w385, new element=w383) -> (w384:dbl[])  [unwired: 1 in]
                      }
                    }
                    n73 = Greater Or Equal?(x=w368, y="Numeric") -> (x >= y?=w377:bool)
                    n74 = case shown="True" w377 {
                      tunnel: [_ TRUE] -> w361
                      tunnel: [0 w401] -> w379
                      tunnel: w378 -> [w393 _]
                      tunnel: w368 -> [_ w399]
                      tunnel: w375 -> [_ w398]
                      tunnel: [_ w396] -> w374
                      frame True {
                        n75 = call "Controller Write PS Filter Enable.vi"("PS Filter Enable"=w393, "Filter Enable"=FALSE) -> ()  [unwired: 13 in, 1 out]
                      }
                      frame False {
                        # "Flush 1-element\nManual Setpoints FIFO"
                        n76 = Increment(x=w399) -> (x+1=w401:i32)
                        n77 = RT FIFO Read(0:w398) -> ()  [unwired: 3 in, 5 out]
                        n78 = feedback #10() -> (w397:u8)  [unwired: 1 in]
                        n79 = case shown="9" w397 {
                          selector: w397 -> [w403 _]
                          tunnel: [w402 u8 5] -> w396
                          frame 0, Default {
                            n80 = Increment(x=w403) -> (x+1=w402:u8)
                          }
                          frame 9 {
                          }
                        }
                        n81 = feedback-in #10(w396) -> ()
                      }
                    }
                    n82 = feedback-in #9(w379) -> ()
                  }
                }
                n83 = Select(t=w312, s=w310, f=u8 0) -> (s? t:f=w311:u8)
              }
            }
            n84 = Replace Array Subset(array=w189, new element #1=w126, new element #2=w124, index #2=w191, new element #3=w123, index #3=w186, new element #4=w192, index #4=w190, new element #5=w178, index #5=w185, new element #6="Missed iteration count", index #6=w184, new element #7="Iteration duration", index #7=w176, new element #8=w173) -> (w187:dbl[])  [unwired: 2 in]
            n85 = RT FIFO Write(0:w181, 1:w187) -> ()  [unwired: 3 in, 4 out]
            n86 = feedback-in #3(w152) -> ()
            n87 = feedback-in #4(w136) -> ()
            n88 = feedback-in #5(w122) -> ()
            n89 = feedback-in #6(w132) -> ()
            n90 = feedback-in #7(w123) -> ()
            n91 = case shown="4" w140 {
              selector: w140 -> [w202 _]
              tunnel: [w201 u8 1] -> w139
              frame 0, Default {
                n92 = Increment(x=w202) -> (x+1=w201:u8)
              }
              frame 4 {
              }
            }
            n93 = call "Controller Write PS Filter Data and Address.vi"("PS ADDR"=w141, "PS DATA"=w142, "Address"=w143, "Data"=w144, "error in"=w146) -> ("error out"=w145:errorcluster)  [unwired: 10 in]
            n94 = Unbundle By Name(w145) -> ("code"=w188:i32)
            n95 = feedback-in #8(w139) -> ()
            n96 = case shown="-2147138393, -2147137765, -66499..-66200, -66099..-66000, 66030" w188 {
              tunnel: w174 -> [_ w233]
              frame 0, Default {
              }
              frame -2147138393, -2147137765, -66499..-66200, -66099..-66000, 66030 {
                w235 = 2 items=["Configuration Mode"=1, "Active Mode"=2] ("mode (Active Mode)")
                w236 = 1 items=["Configuration Mode"=1, "Active Mode"=2] ("mode (Active Mode)")
                # "Restart EtherCAT network on any error on \nScan Engine Warning (66030)\nI/O Scan Driver\t(-66000..-66099) or\nI/O Variables\t(-66200..-66299) or\nNI Scan Engine VIs\t(-66300..-66399) or\nNI Scan Engine (-66400..-66499)\nNetwork Error (-2147138393, -2147137765)"
                n97 = call <vilib>:"Set Scan Engine Mode.vi"("mode (Active Mode)"=w236) -> ("error out"=w237:errorcluster)  [unwired: 14 in]
                n98 = call <vilib>:"Clear All Faults.vi"("error in (no error)"=w237) -> ("error out"=w234:errorcluster)  [unwired: 1 in, 9 out]
                n99 = RT FIFO Write(0:w233, 1:u16 2 ("element")) -> ()  [unwired: 3 in, 4 out]
                n100 = call <vilib>:"Set Scan Engine Mode.vi"("mode (Active Mode)"=w235, "error in (no error)"=w234) -> ()  [unwired: 13 in, 1 out]
              }
            }
            n101 = call <vilib>:"Clear Errors.vi"("error in (no error)"=w145) -> ("error out"=w170:errorcluster)  [unwired: 6 in]
          }
          frame #1 {
          }
        }
      }
      frame True {
        w466 = 3  # Number of Diagnostic Data (Time-Critical Loop)
        # "### Remove 'Use Additional BPM LPF', 'BPM LPF Cutoff', 'Correction Period', 'Request Setpoints Rate' parameters from XML configuration file"
        n102 = Unbundle By Name("FOFB Configuration") -> ("Number of BPM Readings"=w444:i32, "Number of Correctors"=w435:i32, "Number of Actuation Chassis"=w445:i32)
        n103 = Unbundle By Name("PS Variables") -> ("PS Reading Variables"=w454:refnum<k21>[], "PS Status Variables"=w474:refnum<k21>[], "PS Filter Enable"=w438:refnum<k21>[], "PS ADDR"=w439:refnum<k21>[], "PS DATA"=w440:refnum<k21>[], "PS Setpoint Variables"=w473:refnum<k21>[], "PS ON-OFF Variables"=w472:refnum<k21>[])
        n104 = Unbundle By Name("BPM Variables") -> ("BPM Variables"=w475:refnum<k21>[])
        n105 = Unbundle By Name("Sync Objects") -> ("Blocking.Monitoring BPM and PS Data FIFO"=w461:refnum<k33>, "Blocking.PS Manual Setpoints FIFO"=w455:refnum<k33>, "Blocking.FOFB Controller Errors FIFO"=w460:refnum<k33>)
        n106 = Unbundle By Name("Sync Objects") -> ("Non-blocking.Actuation State Change Request FIFO"=w476:refnum<k33>, "Non-blocking.FOFB Variables Queue"=w452:refnum<queue>, "Blocking.BPM and PS Modified Values"=w443:refnum<k33>)
        n107 = Unbundle By Name("FOFB Configuration") -> ()  [unwired: 4 out]
        n108 = Add(x=w444, y=w435) -> (x+y=w470:i32)
        n109 = Unbundle By Name("FOFB Configuration") -> ("FOFB Parameters.Fast Acquisition.Acquisition Period"=w441:u32)
        n110 = Add(x=w470, y=w435) -> (x+y=w469:i32)
        n111 = Add(x=w469, y=w445) -> (x+y=w468:i32)
        n112 = Add(x=w468, y=w445) -> (x+y=w450:i32)
        n113 = Add(x=w450, y=w466) -> (x+y=w451:i32)
        n114 = Initialize Array(u8 127, w445) -> (w459:u8[])
        n115 = call "Controller Extract FOFB Variables.vi"("FOFB Configuration"="FOFB Configuration") -> ("FOFB Variables"=w453:T16)  [unwired: 9 in, 1 out]
        n116 = Lossy Enqueue Element(queue=w452, element=w453) -> ()  [unwired: 1 in, 4 out]
        n117 = Max & Min(x=w435, y=w444) -> (max(x,y)=w447:i32)  [unwired: 1 out]
        n118 = Initialize Array(0.0 ("element"), w451) -> (w471:dbl[])
        n119 = Increment(x=w447) -> (x+1=w446:i32)
        n120 = Initialize Array(0.0, w435) -> (w434:dbl[])
        n121 = disable-structure shown="default" {
          disable-tunnel: [w479 w480 w482] -> w437
          disable-tunnel: w455 -> [w478 _ _]
          disable-tunnel: w454 -> [_ _ w481]
          disable-tunnel: w434 -> [_ w480 _]
          frame condition #0 {
            # "Waits for confirmation of corrector setpoints from OPR1"
            n122 = RT FIFO Read(0:w478, 2:-1 ("timeout in ms (0)")) -> (9:w479:dbl[])  [unwired: 2 in, 4 out]
          }
          frame condition #1 (active) {
          }
          frame condition #2 {
            n123 = call "Controller Average Readings Inputs.vi"("PS Reading Variables"=w481) -> ("PS"=w482:dbl[])  [unwired: 11 in, 3 out]
          }
        }
        n124 = Add(x=w450, y=1) -> (x+y=w456:i32)
        n125 = Initialize Array(sgl 0.0, w446) -> (w448:sgl[])
      }
    }
  }
  "error out" <- w2
